vi "Shifter Controller.vi"(10 "ShiftHigh":bool) -> ()   [LabVIEW 2013]
uses:
  Commands/Shifter-ShiftLow-Cmd/SF-ShiftLow-Cmd.lvclass
  Systems/Shifter/Shifter.lvclass
  Systems/System/System.lvclass
  Commands/Shifter-ShiftHigh-Cmd/SF-ShiftHigh-Cmd.lvclass
  Robot Global Data.vi
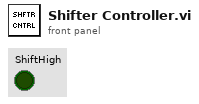
[diagram p1: front panel]
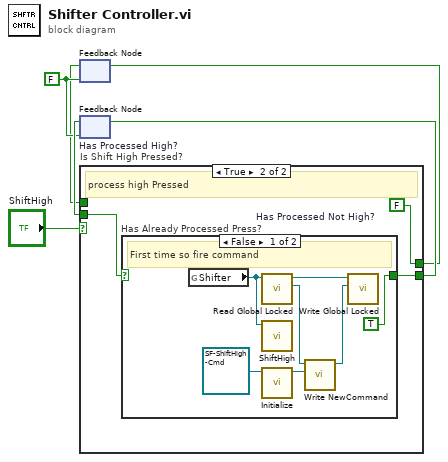
[diagram p0: block diagram]
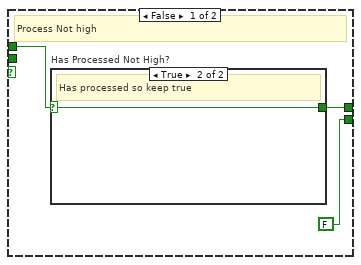
[diagram p2: hidden frame]
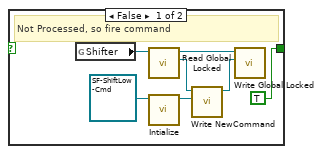
[diagram p3: hidden frame]
diagram:
  w3 = FALSE
  n1 = feedback #1 "Has Processed Not High?"(w3) -> (w2:bool)
  n2 = feedback #2 "Has Processed High?"(w3) -> (w6:bool)
  n3 = case "Is Shift High Pressed?" shown="True" "ShiftHigh" {
    tunnel: w6 -> [_ w20]
    tunnel: [FALSE w19] -> w5
    tunnel: w2 -> [w8 _]
    tunnel: [w7 FALSE] -> w1
    frame False {
      # "Process Not high"
      n4 = case "Has Processed Not High?" shown="True" w8 {
        selector: w8 -> [_ w17]
        tunnel: [TRUE w17] -> w7
        frame False {
          # "Not Processed, so fire command"
          n5 = global read "Robot Global Data.vi" "Shifter"() -> (w12:refnum<class "Shifter.lvclass">)
          n6 = call-dynamic "Read Global Locked.vi"("Shifter in"=w12) -> ("Global"=w16:refnum<class "System.lvclass">, "Shifter out"=w10:refnum<class "Shifter.lvclass">)  [unwired: 7 in, 2 out]
          n7 = call-dynamic "Intialize.vi"("Shifter-ShiftLow-Cmd in"=refnum<class "SF-ShiftLow-Cmd.lvclass"> refnum ("SF-ShiftLow-Cmd.lvclass")) -> ("Shifter-ShiftLow-Cmd out"=w14:refnum<class "SF-ShiftLow-Cmd.lvclass">)  [unwired: 9 in, 1 out]
          n8 = call-dynamic "Write NewCommand.vi"("Command.lvclass"=w14, "System in"=w16) -> ("System out"=w13:refnum<class "System.lvclass">)  [unwired: 8 in, 1 out]
          n9 = call-dynamic "Write Global Locked.vi"("Global"=w13, "Shifter in"=w10) -> ()  [unwired: 8 in, 2 out]
        }
        frame True {
          # "Has processed so keep true"
        }
      }
    }
    frame True {
      # "process high Pressed"
      n10 = case "Has Already Processed Press?" shown="False" w20 {
        selector: w20 -> [_ w28]
        tunnel: [TRUE w28] -> w19
        frame False {
          # "First time so fire command"
          n11 = global read "Robot Global Data.vi" "Shifter"() -> (w21:refnum<class "Shifter.lvclass">)
          n12 = call-dynamic "Read Global Locked.vi"("Shifter in"=w21) -> ("Global"=w27:refnum<class "System.lvclass">, "Shifter out"=w22:refnum<class "Shifter.lvclass">)  [unwired: 7 in, 2 out]
          n13 = call-dynamic "ShiftHigh.vi"("Shifter in"=w21) -> ()  [unwired: 9 in, 2 out]
          n14 = call-dynamic "Initialize.vi"("Shifter-ShiftHigh-Cmd in"=refnum<class "SF-ShiftHigh-Cmd.lvclass"> refnum ("SF-ShiftHigh-Cmd.lvclass")) -> ("Shifter-ShiftHigh-Cmd out"=w25:refnum<class "SF-ShiftHigh-Cmd.lvclass">)  [unwired: 9 in, 1 out]
          n15 = call-dynamic "Write NewCommand.vi"("Command.lvclass"=w25, "System in"=w27) -> ("System out"=w24:refnum<class "System.lvclass">)  [unwired: 8 in, 1 out]
          n16 = call-dynamic "Write Global Locked.vi"("Global"=w24, "Shifter in"=w22) -> ()  [unwired: 8 in, 2 out]
        }
        frame True {
          # "Already processed so keep True"
        }
      }
    }
  }
  n17 = feedback-in #1(w1) -> ()
  n18 = feedback-in #2(w5) -> ()
